vi "Compute Distance To Coral.vi"(6 "Target Width (in)":dbl=6.5 format="%.1f", 8 "results":T1, 10 "FOV":dbl=68.5, 11 "Image Src":T2) -> (0 "results out":T1, 1 "Off Angle":dbl, 2 "Raw Coral DIstance":dbl, 3 "Image Dst Out":T2, 4 "Distance":dbl)   [LabVIEW 2023]
doc: "Using the camera lens information and the real world size of the target, use trig and ratios to determine the distance to the target. Also returns the location relative to the image center in a (-1 , 1) coordinate system that may be useful for steering the robot."
uses:
  <vilib>/vision/Image Controls.llb/IMAQ Image.ctl
  Target Fields.ctl
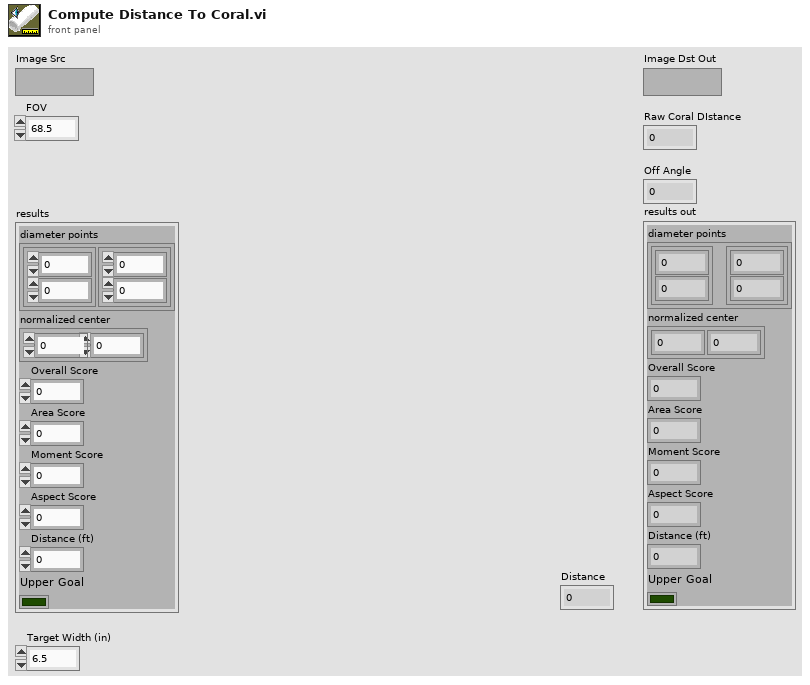
[diagram p1: front panel]
types:
  T1 = typedef "Target Fields.ctl" = cluster{"diameter points":cluster{"first point":cluster{"x":dbl, "y":dbl}, "projected point":cluster{"x":dbl, "y":dbl}}, "normalized center":cluster{"x":dbl, "y":dbl}, "Overall Score":dbl, "Area Score":dbl, "Moment Score":dbl, "Aspect Score":dbl, "Distance (ft)":dbl, "Upper Goal":bool}
  T2 = typedef "IMAQ Image.ctl" = refnum<image>
  T3 = cluster{"first point":cluster{"x":dbl, "y":dbl}, "projected point":cluster{"x":dbl, "y":dbl}}
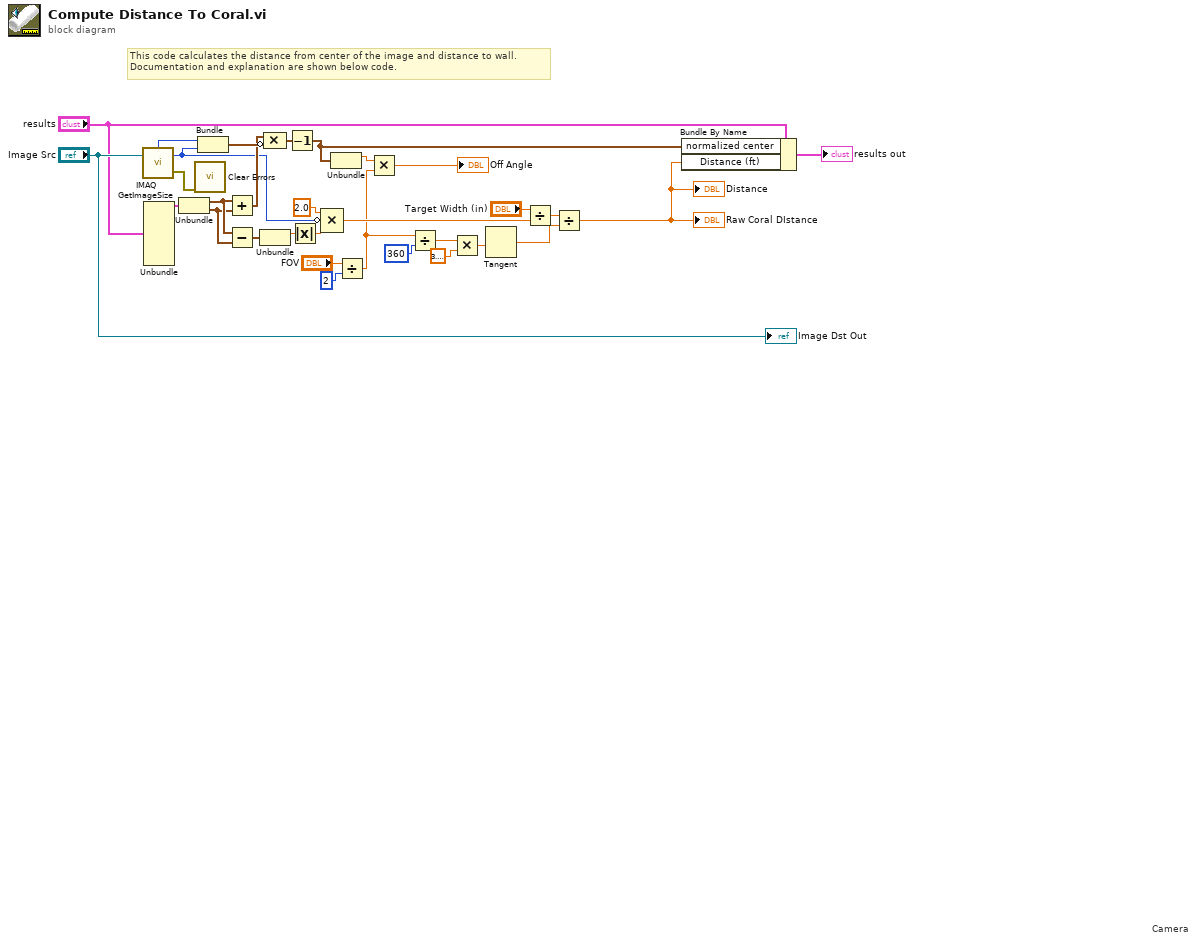
[diagram p0: block diagram]
diagram:
  # "Camera"
  # "This code calculates the distance from center of the image and distance to wall.\nDocumentation and explanation are shown below code."
  n1 = call "IMAQ GetImageSize"("Image"="Image Src") -> ("Y Resolution"=w11:i32, "X Resolution"=w8:i32, "error out"=w23:errorcluster)  [unwired: 3 in]
  n2 = Unbundle("results") -> ("diameter points"=w16:T3)  [unwired: 7 out]
  n3 = Unbundle(w16) -> ("first point"=w14:cluster{"x":dbl, "y":dbl}, "projected point"=w13:cluster{"x":dbl, "y":dbl})
  n4 = call <vilib>:"Clear Errors.vi"("error in (no error)"=w23) -> ()  [unwired: 5 in, 2 out]
  n5 = Bundle("X Resolution"=w8, "Y Resolution"=w11) -> (w15:cluster{"X Resolution":i32, "Y Resolution":i32})  [unwired: 1 in]
  n6 = Add(x=w14, y=w13) -> (x+y=w12:cluster{"x":dbl, "y":dbl})
  n7 = Subtract(x=w14, y=w13) -> (x-y=w20:cluster{"x":dbl, "y":dbl})
  n8 = Unbundle(w20) -> ("x"=w19:dbl)  [unwired: 1 out]
  n9 = Compound Arithmetic op=MULTIPLY(w12, invert w15) -> (w3:cluster{dbl, dbl})
  n10 = Decrement(x=w3) -> (x-1=w9:cluster{dbl, dbl})
  n11 = Absolute Value(x=w19) -> (abs(x)=w21:dbl)
  n12 = Compound Arithmetic op=MULTIPLY(2.0, invert w11, w21) -> (w24:dbl)
  n13 = Unbundle(w9) -> (w7:dbl)  [unwired: 1 out]
  n14 = Divide(x="FOV", y=2) -> (x/y=w2:dbl)
  n15 = Multiply(x=w7, y=w2) -> (x*y=→"Off Angle":dbl)
  n16 = Divide(x=w2, y=360) -> (x/y=w28:dbl)
  n17 = Multiply(x=w28, y=3.141592653589793) -> (x*y=w29:dbl)
  n18 = Tangent(1:w29) -> (0:w26:dbl)
  n19 = Divide(x="Target Width (in)", y=w24) -> (x/y=w6:dbl)
  n20 = Divide(x=w6, y=w26) -> (x/y=w5:dbl)
  "Raw Coral DIstance" <- w5
  "Distance" <- w5
  n21 = Bundle By Name(cluster="results", "normalized center"=w9, "Distance (ft)"=w5) -> (→"results out":T1)
  "Image Dst Out" <- "Image Src"
